vi "MyFPGACode.vi"() -> ()   [LabVIEW 2012, in "MyFPGACode.lvlib"]
doc: "This VI was generated automatically using the FPGA Wizard. You can modify the VI normally."
uses:
  MyFPGACode.lvlib
  <vilib>/Platform/TimedLoop/XDataNode/timing_clust.ctl
  <vilib>/Platform/TimedLoop/XDataNode/nitl_modes.ctl
  <vilib>/Platform/TimedLoop/XDataNode/wakeup.ctl
  <vilib>/rvi/Emulation/niFpgaSctlEmulationGetInTimedLoop.vi
  <vilib>/rvi/Emulation/niFpgaSctlEmulationGlobalWrite.vi
  <vilib>/rvi/Emulation/niFpgaSctlEmulationRegisterWithScheduler.vi
  <vilib>/rvi/Emulation/niFpgaSctlEmulationScheduler.vi
  <vilib>/rvi/eio/common/nirviEmuTemplateMethod_errors.vi
  <vilib>/Platform/TimedLoop/XDataNode/XDataNode.xnode
  <vilib>/eio/EIONode/EIONode.xnode
  <vilib>/Platform/TimedLoop/XDataNode/XDNodeRunTimeDep.lvlib
panel:
  in  "Direction J2":bool
  in  "_Direction J2":bool
  in  "PWM Settings (Port0/DIO5)":cluster{"ActiveTime":u32, "Period":u32}
  in  "_PWM Settings (Port0/DIO5)":cluster{"ActiveTime":u32, "Period":u32}
  out "AI (ModA/AI0)":fxp<+/-,26,5> format="%.23g"
  in  "Local Stop 0":bool
  out "Data Ready 0":bool
  in  "Start 0":bool
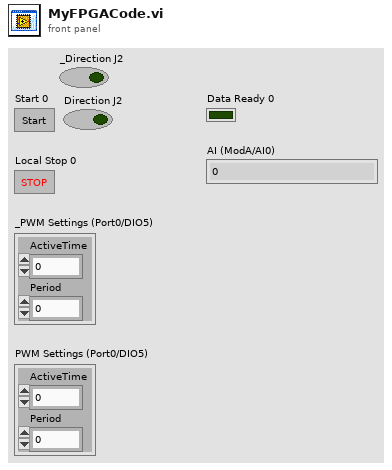
[diagram p1: front panel]
types:
  T1 = typedef "XDNodeRunTimeDep.lvlib/timing_clust.ctl" = cluster{"Expected End [f-1]":u64, "Actual End [f-1]":u64, "Finished Late? [f-1]":bool, "Expected End [i-1]":u64, "Actual End [i-1]":u64, "Finished Late? [i-1]":bool, "Expected Start [i]":u64, "Actual Start [i]":u64, "Expected Start [f]":u64, "Actual Start [f]":u64, "Source Name":string, "Structure Name":string, "Period":i64, "Deadline":i64, "Offset":i64, "Start":i64, "Priority":i32, "Timeout":i32, "Mode":T2, "Wakeup Reason":T3, "Error":errorcluster, "Source Type":string, "Secondary Source Type":string, "Global End Time":u64, "Global Start Time":u64, "Frame Duration":u64, "Iteration Duration":u64, "Assigned CPU":i32, "I/O Scan Engine Mode":u32}
  T2 = typedef "XDNodeRunTimeDep.lvlib/nitl_modes.ctl" = enum32{"No Change", "Process missed periods, maintain original phase", "Discard missed periods, maintain original phase", "Process missed periods, ignore original phase", "Discard missed periods, ignore original phase"}
  T3 = typedef "XDNodeRunTimeDep.lvlib/wakeup.ctl" = enum32{"Normal", "Aborted", "Asynchronous wakeup", "Timing source error", "Timed loop error", "Timeout"}
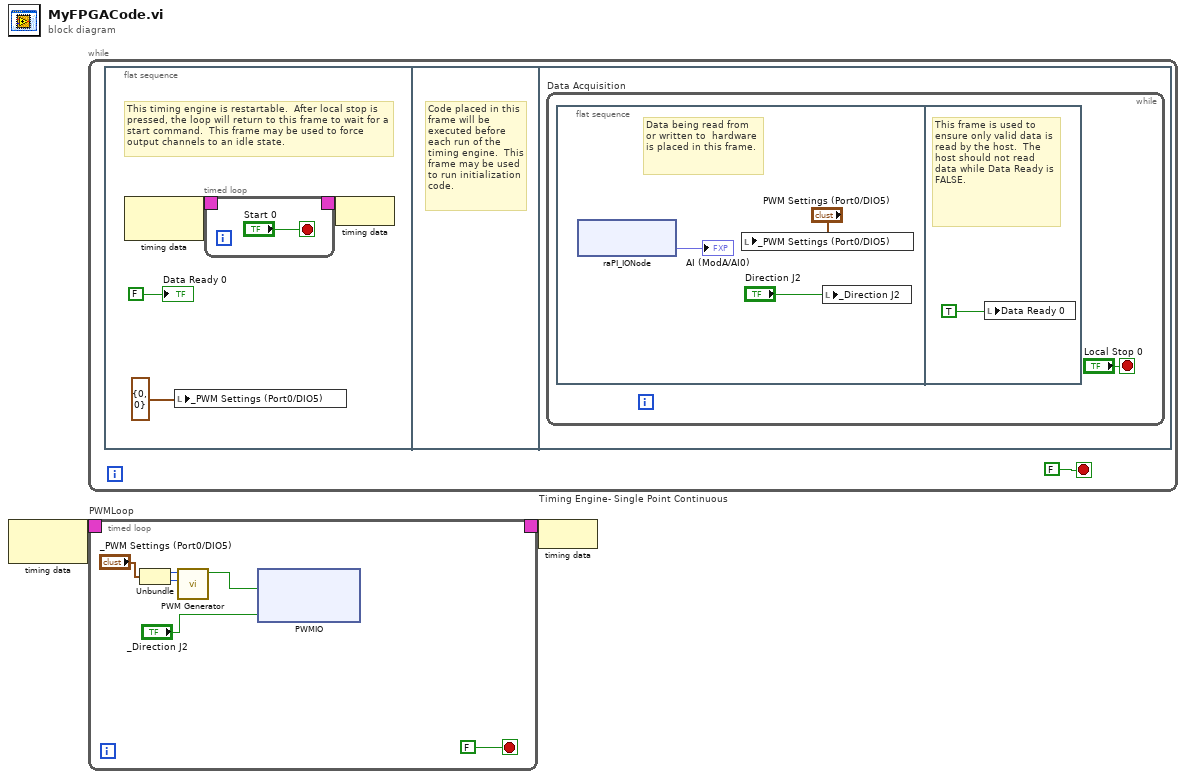
[diagram p0: block diagram]
diagram:
  n1 = node-c288 ("Input Node")() -> (w2:T1)  [unwired: 1 in]
  n2 = while "Timing Engine- Single Point Continuous" {
    stop <- FALSE stop-if-true
    n3 = flat-sequence "MainSeq" {
      frame #0 {
        # "This timing engine is restartable.  After local stop is pressed, the loop will return to this frame to wait for a start command.  This frame may be used to force output channels to an idle state."
        n4 = node-c288 ("Input Node")() -> (w6:T1)  [unwired: 1 out]
        n5 = local write "_PWM Settings (Port0/DIO5)"(cluster{"ActiveTime":u32, "Period":u32} {"ActiveTime"=0, "Period"=0} ("ToPWM Parameters")) -> ()
        n6 = timed-loop "initWait" {
          timing: w6 -> [_]
          timing-out: [_] -> w5
          stop <- "Start 0" stop-if-true
        }
        n7 = node-c288 ("Output Node")(w5) -> ()
        "Data Ready 0" <- FALSE
      }
      frame #1 {
        # "Code placed in this frame will be executed before each run of the timing engine.  This frame may be used to run initialization code."
      }
      frame #2 {
        n8 = while "Data Acquisition" {
          stop <- "Local Stop 0" stop-if-true
          n9 = flat-sequence "Data Acquisition Sequence" {
            frame #0 {
              # "Data being read from or written to  hardware is placed in this frame."
              n10 = xnode ("raPI_IONode")() -> ("ModA/AI0"=→"AI (ModA/AI0)":fxp<+/-,26,5>)  [unwired: 1 in, 1 out]
              n11 = local write "_PWM Settings (Port0/DIO5)"("PWM Settings (Port0/DIO5)") -> ()
              n12 = local write "_Direction J2"("Direction J2") -> ()
            }
            frame #1 {
              # "This frame is used to ensure only valid data is read by the host.  The host should not read data while Data Ready is FALSE."
              n13 = local write "Data Ready 0"(TRUE) -> ()
            }
          }
        }
      }
    }
  }
  n14 = timed-loop "PWMLoop" {
    timing: w2 -> [_]
    timing-out: [_] -> w1
    stop <- FALSE stop-if-true
    n15 = Unbundle("_PWM Settings (Port0/DIO5)") -> ("ActiveTime"=w20:u32, "Period"=w19:u32)
    n16 = call "PWM Generator.vi"("Period"=w19, "Active Time"=w20) -> ("Output"=w23:bool)  [unwired: 9 in]
    n17 = xnode ("PWMIO")("Port8/DIO5"=w23, "Port8/DIO6"="_Direction J2") -> ()  [unwired: 2 in, 2 out]
  }
  n18 = node-c288 ("Output Node")(w1) -> ()
